vi "SaveImage.vi"(11 "Refnum in":T1) -> ()   [LabVIEW 2017]
uses:
  <vilib>/vision/Image Controls.llb/IMAQ Image.ctl
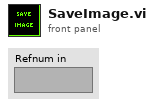
[diagram p1: front panel]
types:
  T1 = typedef "IMAQ Image.ctl" = refnum<image>
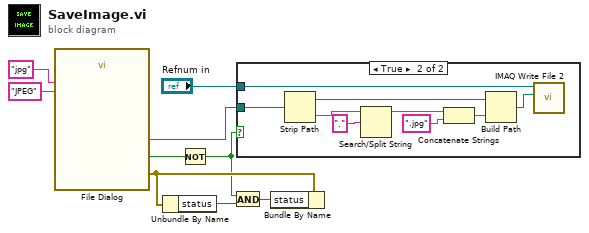
[diagram p0: block diagram]
diagram:
  n1 = call "File Dialog"("pattern (all files)"="jpg", "pattern label"="JPEG") -> ("selected path"=w8:path, "cancelled"=w5:bool, "error out"=w4:errorcluster)  [unwired: 10 in, 1 out]
  n2 = Unbundle By Name(w4) -> ("status"=w1:bool)
  n3 = Not(x=w5) -> (.not. x?=w2:bool)
  n4 = And(x=w2, y=w1) -> (x .and. y?=w3:bool)
  n5 = case shown="True" w2 {
    tunnel: "Refnum in" -> [_ w18]
    tunnel: w8 -> [_ w10]
    frame False {
    }
    frame True {
      n6 = Strip Path(path=w10) -> (stripped path=w11:path, name=w12:string)
      n7 = Search/Split String(string=w12, search string/char (-)=".") -> (substring before match=w14:string)  [unwired: 1 in, 2 out]
      n8 = Concatenate Strings(w14, ".jpg" ("string")) -> (w16:string)
      n9 = Build Path(base path=w11, name or relative path=w16) -> (appended path=w17:path)
      n10 = call-poly "IMAQ Write File 2"("File Path"=w17, "Image"=w18) -> ()  [unwired: 8 in, 2 out]
    }
  }
  n11 = Bundle By Name(cluster=w4, "status"=w3) -> ()  [unwired: 1 out]
